vi "XML_Get_Modbus_Items.vi"(8 "error in (no error)":errorcluster, 10 "General Settings":T1={"Communication_Type"=0, "Modbus_Type"=0, "Read_Write_Loop_Period"=-1, "TCP Settings"={"TCP_Settings_Port"=0, "TCP_Settings_IP_Timeout"=0, "TCP_Settings_IP_Slave_Address"=""}, "Serial Settings"={"Serial_Settings_Flow_Control"=0, "Serial_Settings_Baud_Rate"=0, "Serial_Settings_Parity"=0, "Serial_Settings_Resource_Name"="", "Serial_Settings_Serial_Type"=0, "Serial_Settings_Unit_ID"=0}} {"Communication_Type" items=["TCP", "Serial"]; "Modbus_Type" items=["Master", "Slave"]; "Serial Settings"."Serial_Settings_Flow_Control" items=["None", "XONXOFF", "RTSCTS", "XONXOFFANDRTSCTS", "DTRDSR", "XONXOFFANDDTRDSR"]; "Serial Settings"."Serial_Settings_Parity" items=["None", "Odd", "Even"]; "Serial Settings"."Serial_Settings_Serial_Type" items=["RTU", "ASCII"]}, 11 "reference out":refnum<k24>) -> (0 "error out":errorcluster, 2 "Array":T7[](array[typedef]), 3 "reference out":refnum<k24>)   [LabVIEW 2014, in "XML_Deserializer.lvlib"]
uses:
  XML_Deserializer.lvlib
  C:/Users/vruault.AMER/Desktop/Source code/XML Deserializer/XML VIs/API/Sub-VIs/Modbus_CD_XML.dll
  Modbus_CD_XML.dll
  Controls/Modbus_Items.ctl
  Controls/Modbus_Item_Type.ctl
  Controls/Modbus_General_Settings.ctl
  Controls/Modbus_Communication_Type.ctl
  Controls/Modbus_Type.ctl
  Controls/Modbus_Serial_Settings_Flow_Control.ctl
  Controls/Modbus_Serial_Settings_Parity.ctl
  Controls/Modbus_Serial_Settings_Serial_Type.ctl
  Shared/Modbus Shared.lvlib
  System Explorer/Modbus System Explorer.lvlib
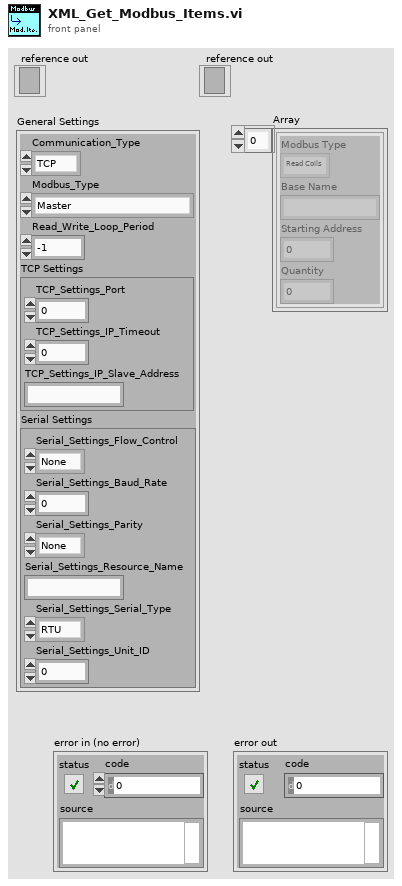
[diagram p1: front panel]
types:
  T1 = typedef "Modbus Shared.lvlib/Modbus_General_Settings.ctl" = cluster{"Communication_Type":T2, "Modbus_Type":T3, "Read_Write_Loop_Period":i64, "TCP Settings":cluster{"TCP_Settings_Port":u16, "TCP_Settings_IP_Timeout":u32, "TCP_Settings_IP_Slave_Address":string}, "Serial Settings":cluster{"Serial_Settings_Flow_Control":T4, "Serial_Settings_Baud_Rate":u32, "Serial_Settings_Parity":T5, "Serial_Settings_Resource_Name":string, "Serial_Settings_Serial_Type":T6, "Serial_Settings_Unit_ID":u8}}
  T2 = typedef "Modbus Shared.lvlib/Modbus_Communication_Type.ctl" = i32
  T3 = typedef "Modbus Shared.lvlib/Modbus_Type.ctl" = i32
  T4 = typedef "Modbus Shared.lvlib/Modbus_Serial_Settings_Flow_Control.ctl" = i32
  T5 = typedef "Modbus Shared.lvlib/Modbus_Serial_Settings_Parity.ctl" = i32
  T6 = typedef "Modbus Shared.lvlib/Modbus_Serial_Settings_Serial_Type.ctl" = i32
  T7 = typedef "Modbus Shared.lvlib/Modbus_Items.ctl" = cluster{"Modbus Type":T8, "Base Name":string, "Starting Address":u16, "Quantity":u16}
  T8 = typedef "Modbus Shared.lvlib/Modbus_Item_Type.ctl" = enum16{"Read Coils", "Read Discrete Inputs", "Read Holding Registers", "Read Input Registers", "Write Multiple Coils", "Write Multiple Holding Registers", "Write Single Coil", "Write Single Holding Register", "Write Multiple Discrete Inputs", "Write Multiple Input Registers"}
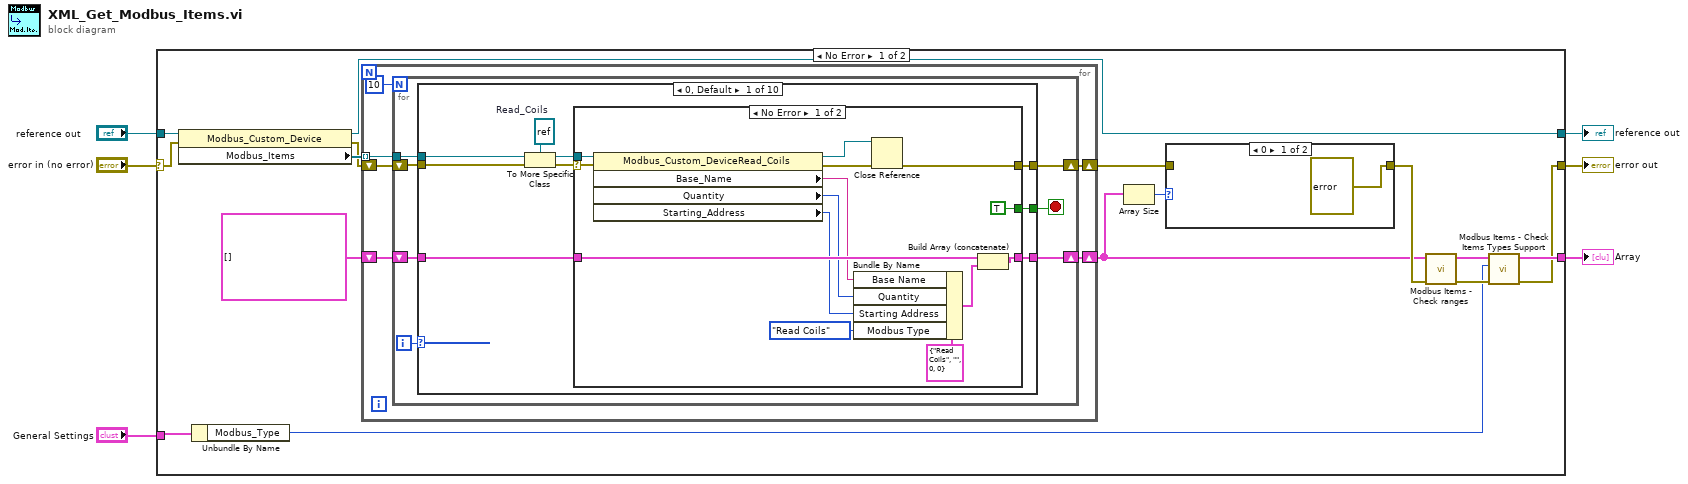
[diagram p0: block diagram]
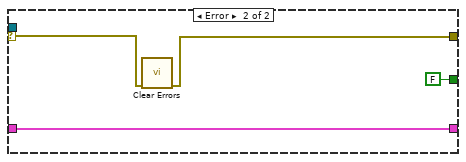
[diagram p3: hidden frame]
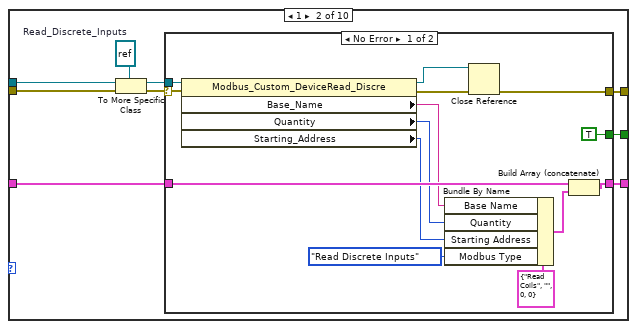
[diagram p4: hidden frame]
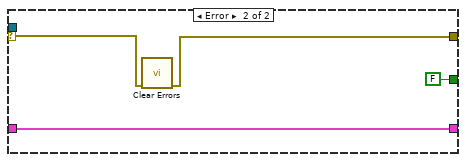
[diagram p5: hidden frame]
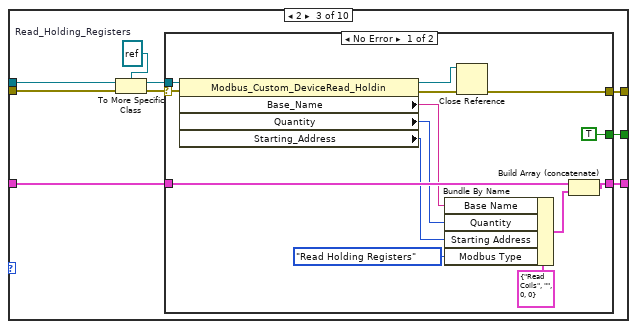
[diagram p6: hidden frame]
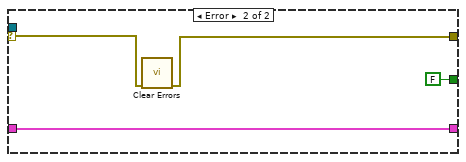
[diagram p7: hidden frame]
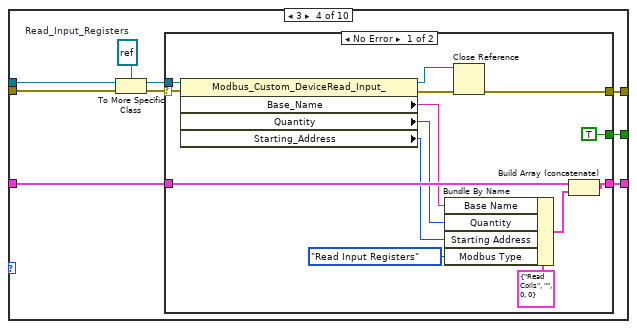
[diagram p8: hidden frame]
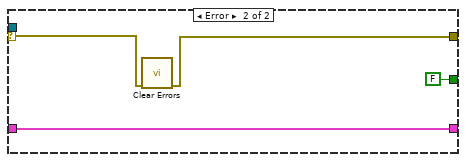
[diagram p9: hidden frame]
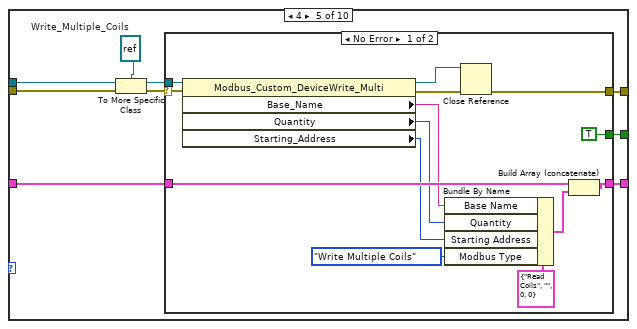
[diagram p10: hidden frame]
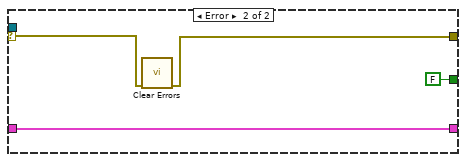
[diagram p11: hidden frame]
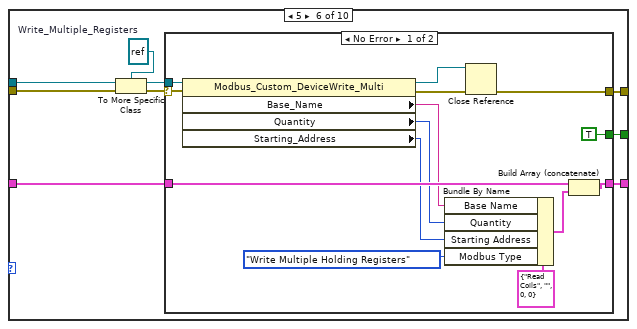
[diagram p12: hidden frame]
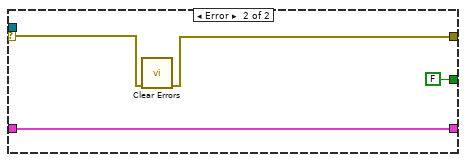
[diagram p13: hidden frame]
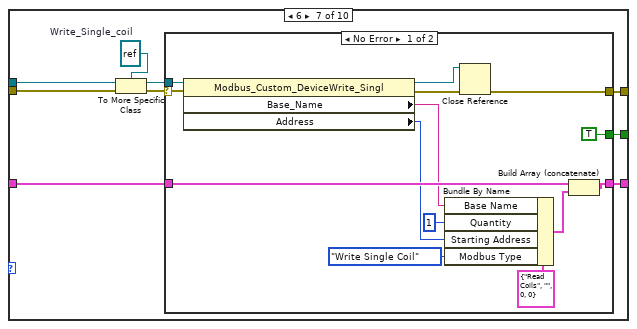
[diagram p14: hidden frame]
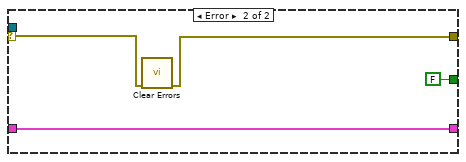
[diagram p15: hidden frame]
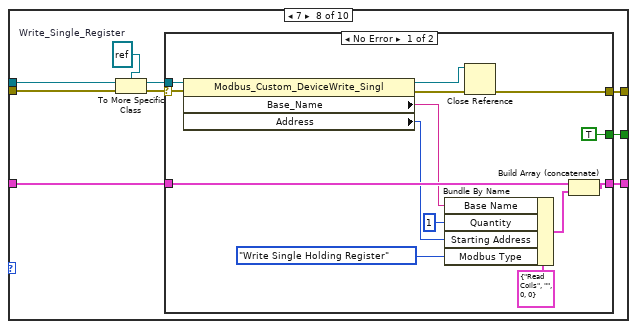
[diagram p16: hidden frame]
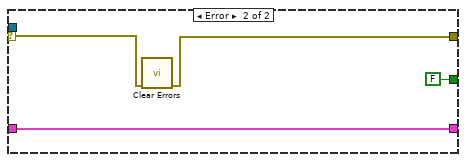
[diagram p17: hidden frame]
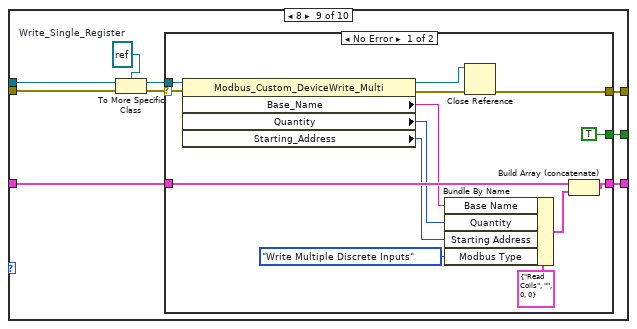
[diagram p18: hidden frame]
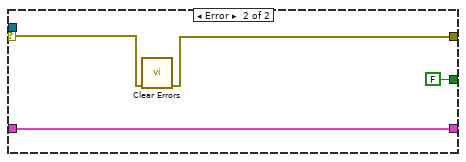
[diagram p19: hidden frame]
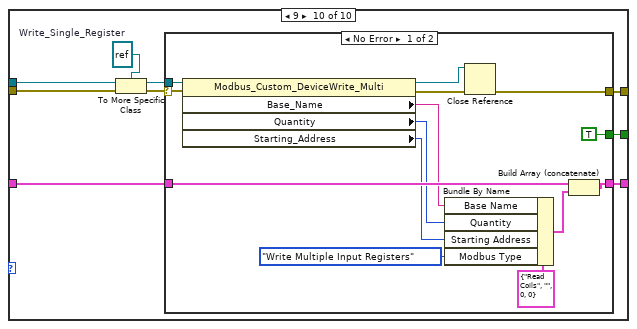
[diagram p20: hidden frame]
diagram:
  n1 = case shown="No Error" "error in (no error)" {
    selector: "error in (no error)" -> [w18 w310]
    tunnel: [w10 T7[] []] -> w2
    tunnel: [w9 w310] -> w3
    tunnel: "reference out" -> [w19 w308]
    tunnel: [w17 w308] -> w6
    tunnel: "General Settings" -> [w8 _]
    frame No Error {
      n2 = property class="Modbus_Custom_Device"(reference=w19, error in=w18) -> (reference out=w17:refnum<k24>, error out=w20:errorcluster, "Modbus_Items"=w22:refnum<k24>[])
      n3 = Unbundle By Name(w8) -> ("Modbus_Type"=w7:T3)
      n4 = for {
        tunnel: w22 -> [w30] mode=indexing
        shift-right: [w28] -> w13
        shift-left: T7[] [] -> [w29]
        shift-right: [w27] -> w15
        shift-left: w20 -> [w26]
        n5 = for {
          N: 10 -> [_]
          tunnel: w30 -> [w37]
          shift-right: [w33] -> w28
          shift-left: w29 -> [w34]
          shift-right: [w32] -> w27
          shift-left: w26 -> [w36]
          i -> [w35]
          stop <- w31 stop-if-true
          n6 = case shown="0, Default" w35 {
            tunnel: w37 -> [w46 w73 w100 w127 w154 w181 w208 w235 w262 w289]
            tunnel: w36 -> [w45 w72 w99 w126 w153 w180 w207 w234 w261 w288]
            tunnel: w34 -> [w41 w69 w96 w123 w150 w177 w204 w231 w258 w285]
            tunnel: [w40 w68 w95 w122 w149 w176 w203 w230 w257 w284] -> w33
            tunnel: [w39 w67 w94 w121 w148 w175 w202 w229 w256 w283] -> w32
            tunnel: [w38 w66 w93 w120 w147 w174 w201 w228 w255 w282] -> w31
            frame 0, Default {
              w44 = refnum<k24> refnum  # Read_Coils
              n7 = To More Specific Class(target class=w44, reference=w46, error in=w45) -> (specific class reference=w43:refnum<k24>, error out=w42:errorcluster)
              n8 = case shown="No Error" w42 {
                selector: w42 -> [w59 w64]
                tunnel: w43 -> [w60 _]
                tunnel: w41 -> [w57 w61]
                tunnel: [w56 w61] -> w40
                tunnel: [w48 w62] -> w39
                tunnel: [TRUE FALSE] -> w38
                frame No Error {
                  n9 = property class="Modbus_Custom_DeviceRead_Coils"(reference=w60, error in=w59) -> (reference out=w47:refnum<k24>, error out=w49:errorcluster, "Base_Name"=w52:string, "Quantity"=w51:u16, "Starting_Address"=w50:u16)
                  n10 = Bundle By Name(cluster=T7 {"Modbus Type"=enum."Read Coils", "Base Name"="", "Starting Address"=0, "Quantity"=0} ("Modbus Items"), "Base Name"=w52, "Quantity"=w51, "Starting Address"=w50, "Modbus Type"=Modbus_Item_Type."Read Coils") -> (w55:T7)
                  n11 = Close Reference(reference=w47, error in (no error)=w49) -> (error out=w48:errorcluster)
                  n12 = Build Array (concatenate)(w57, w55) -> (w56:T7[])
                }
                frame Error {
                  n13 = call <vilib>:"Clear Errors.vi"("error in (no error)"=w64) -> ("error out"=w62:errorcluster)  [unwired: 5 in, 1 out]
                }
              }
            }
            frame 1 {
              w65 = refnum<k24> refnum  # Read_Discrete_Inputs
              n14 = To More Specific Class(target class=w65, reference=w73, error in=w72) -> (specific class reference=w71:refnum<k24>, error out=w70:errorcluster)
              n15 = case shown="No Error" w70 {
                selector: w70 -> [w86 w91]
                tunnel: w71 -> [w87 _]
                tunnel: w69 -> [w84 w88]
                tunnel: [w83 w88] -> w68
                tunnel: [w74 w89] -> w67
                tunnel: [TRUE FALSE] -> w66
                frame No Error {
                  n16 = property class="Modbus_Custom_DeviceRead_Discre"(reference=w87, error in=w86) -> (reference out=w76:refnum<k24>, error out=w75:errorcluster, "Base_Name"=w79:string, "Quantity"=w78:u16, "Starting_Address"=w77:u16)
                  n17 = Bundle By Name(cluster=T7 {"Modbus Type"=enum."Read Coils", "Base Name"="", "Starting Address"=0, "Quantity"=0} ("Modbus Items"), "Base Name"=w79, "Quantity"=w78, "Starting Address"=w77, "Modbus Type"=Modbus_Item_Type."Read Discrete Inputs") -> (w82:T7)
                  n18 = Close Reference(reference=w76, error in (no error)=w75) -> (error out=w74:errorcluster)
                  n19 = Build Array (concatenate)(w84, w82) -> (w83:T7[])
                }
                frame Error {
                  n20 = call <vilib>:"Clear Errors.vi"("error in (no error)"=w91) -> ("error out"=w89:errorcluster)  [unwired: 5 in, 1 out]
                }
              }
            }
            frame 2 {
              w92 = refnum<k24> refnum  # Read_Holding_Registers
              n21 = To More Specific Class(target class=w92, reference=w100, error in=w99) -> (specific class reference=w98:refnum<k24>, error out=w97:errorcluster)
              n22 = case shown="No Error" w97 {
                selector: w97 -> [w113 w118]
                tunnel: w98 -> [w114 _]
                tunnel: w96 -> [w111 w115]
                tunnel: [w110 w115] -> w95
                tunnel: [w101 w116] -> w94
                tunnel: [TRUE FALSE] -> w93
                frame No Error {
                  n23 = property class="Modbus_Custom_DeviceRead_Holdin"(reference=w114, error in=w113) -> (reference out=w103:refnum<k24>, error out=w102:errorcluster, "Base_Name"=w106:string, "Quantity"=w105:u16, "Starting_Address"=w104:u16)
                  n24 = Bundle By Name(cluster=T7 {"Modbus Type"=enum."Read Coils", "Base Name"="", "Starting Address"=0, "Quantity"=0} ("Modbus Items"), "Base Name"=w106, "Quantity"=w105, "Starting Address"=w104, "Modbus Type"=Modbus_Item_Type."Read Holding Registers") -> (w109:T7)
                  n25 = Close Reference(reference=w103, error in (no error)=w102) -> (error out=w101:errorcluster)
                  n26 = Build Array (concatenate)(w111, w109) -> (w110:T7[])
                }
                frame Error {
                  n27 = call <vilib>:"Clear Errors.vi"("error in (no error)"=w118) -> ("error out"=w116:errorcluster)  [unwired: 5 in, 1 out]
                }
              }
            }
            frame 3 {
              w119 = refnum<k24> refnum  # Read_Input_Registers
              n28 = To More Specific Class(target class=w119, reference=w127, error in=w126) -> (specific class reference=w125:refnum<k24>, error out=w124:errorcluster)
              n29 = case shown="No Error" w124 {
                selector: w124 -> [w140 w145]
                tunnel: w125 -> [w141 _]
                tunnel: w123 -> [w138 w142]
                tunnel: [w137 w142] -> w122
                tunnel: [w128 w143] -> w121
                tunnel: [TRUE FALSE] -> w120
                frame No Error {
                  n30 = property class="Modbus_Custom_DeviceRead_Input_"(reference=w141, error in=w140) -> (reference out=w130:refnum<k24>, error out=w129:errorcluster, "Base_Name"=w133:string, "Quantity"=w132:u16, "Starting_Address"=w131:u16)
                  n31 = Bundle By Name(cluster=T7 {"Modbus Type"=enum."Read Coils", "Base Name"="", "Starting Address"=0, "Quantity"=0} ("Modbus Items"), "Base Name"=w133, "Quantity"=w132, "Starting Address"=w131, "Modbus Type"=Modbus_Item_Type."Read Input Registers") -> (w136:T7)
                  n32 = Close Reference(reference=w130, error in (no error)=w129) -> (error out=w128:errorcluster)
                  n33 = Build Array (concatenate)(w138, w136) -> (w137:T7[])
                }
                frame Error {
                  n34 = call <vilib>:"Clear Errors.vi"("error in (no error)"=w145) -> ("error out"=w143:errorcluster)  [unwired: 5 in, 1 out]
                }
              }
            }
            frame 4 {
              w146 = refnum<k24> refnum  # Write_Multiple_Coils
              n35 = To More Specific Class(target class=w146, reference=w154, error in=w153) -> (specific class reference=w152:refnum<k24>, error out=w151:errorcluster)
              n36 = case shown="No Error" w151 {
                selector: w151 -> [w167 w172]
                tunnel: w152 -> [w168 _]
                tunnel: w150 -> [w165 w169]
                tunnel: [w164 w169] -> w149
                tunnel: [w156 w170] -> w148
                tunnel: [TRUE FALSE] -> w147
                frame No Error {
                  n37 = property class="Modbus_Custom_DeviceWrite_Multi"(reference=w168, error in=w167) -> (reference out=w155:refnum<k24>, error out=w157:errorcluster, "Base_Name"=w160:string, "Quantity"=w159:u16, "Starting_Address"=w158:u16)
                  n38 = Bundle By Name(cluster=T7 {"Modbus Type"=enum."Read Coils", "Base Name"="", "Starting Address"=0, "Quantity"=0} ("Modbus Items"), "Base Name"=w160, "Quantity"=w159, "Starting Address"=w158, "Modbus Type"=Modbus_Item_Type."Write Multiple Coils") -> (w163:T7)
                  n39 = Close Reference(reference=w155, error in (no error)=w157) -> (error out=w156:errorcluster)
                  n40 = Build Array (concatenate)(w165, w163) -> (w164:T7[])
                }
                frame Error {
                  n41 = call <vilib>:"Clear Errors.vi"("error in (no error)"=w172) -> ("error out"=w170:errorcluster)  [unwired: 5 in, 1 out]
                }
              }
            }
            frame 5 {
              w173 = refnum<k24> refnum  # Write_Multiple_Registers
              n42 = To More Specific Class(target class=w173, reference=w181, error in=w180) -> (specific class reference=w179:refnum<k24>, error out=w178:errorcluster)
              n43 = case shown="No Error" w178 {
                selector: w178 -> [w194 w199]
                tunnel: w179 -> [w195 _]
                tunnel: w177 -> [w192 w196]
                tunnel: [w191 w196] -> w176
                tunnel: [w182 w197] -> w175
                tunnel: [TRUE FALSE] -> w174
                frame No Error {
                  n44 = property class="Modbus_Custom_DeviceWrite_Multi"(reference=w195, error in=w194) -> (reference out=w183:refnum<k24>, error out=w184:errorcluster, "Base_Name"=w187:string, "Quantity"=w186:u16, "Starting_Address"=w185:u16)
                  n45 = Bundle By Name(cluster=T7 {"Modbus Type"=enum."Read Coils", "Base Name"="", "Starting Address"=0, "Quantity"=0} ("Modbus Items"), "Base Name"=w187, "Quantity"=w186, "Starting Address"=w185, "Modbus Type"=Modbus_Item_Type."Write Multiple Holding Registers") -> (w190:T7)
                  n46 = Close Reference(reference=w183, error in (no error)=w184) -> (error out=w182:errorcluster)
                  n47 = Build Array (concatenate)(w192, w190) -> (w191:T7[])
                }
                frame Error {
                  n48 = call <vilib>:"Clear Errors.vi"("error in (no error)"=w199) -> ("error out"=w197:errorcluster)  [unwired: 5 in, 1 out]
                }
              }
            }
            frame 6 {
              w200 = refnum<k24> refnum  # Write_Single_coil
              n49 = To More Specific Class(target class=w200, reference=w208, error in=w207) -> (specific class reference=w206:refnum<k24>, error out=w205:errorcluster)
              n50 = case shown="No Error" w205 {
                selector: w205 -> [w221 w226]
                tunnel: w206 -> [w222 _]
                tunnel: w204 -> [w219 w223]
                tunnel: [w218 w223] -> w203
                tunnel: [w209 w224] -> w202
                tunnel: [TRUE FALSE] -> w201
                frame No Error {
                  n51 = property class="Modbus_Custom_DeviceWrite_Singl"(reference=w222, error in=w221) -> (reference out=w211:refnum<k24>, error out=w210:errorcluster, "Base_Name"=w214:string, "Address"=w213:u16)
                  n52 = Bundle By Name(cluster=T7 {"Modbus Type"=enum."Read Coils", "Base Name"="", "Starting Address"=0, "Quantity"=0} ("Modbus Items"), "Base Name"=w214, "Quantity"=u16 1, "Starting Address"=w213, "Modbus Type"=Modbus_Item_Type."Write Single Coil") -> (w217:T7)
                  n53 = Close Reference(reference=w211, error in (no error)=w210) -> (error out=w209:errorcluster)
                  n54 = Build Array (concatenate)(w219, w217) -> (w218:T7[])
                }
                frame Error {
                  n55 = call <vilib>:"Clear Errors.vi"("error in (no error)"=w226) -> ("error out"=w224:errorcluster)  [unwired: 5 in, 1 out]
                }
              }
            }
            frame 7 {
              w227 = refnum<k24> refnum  # Write_Single_Register
              n56 = To More Specific Class(target class=w227, reference=w235, error in=w234) -> (specific class reference=w233:refnum<k24>, error out=w232:errorcluster)
              n57 = case shown="No Error" w232 {
                selector: w232 -> [w248 w253]
                tunnel: w233 -> [w249 _]
                tunnel: w231 -> [w246 w250]
                tunnel: [w245 w250] -> w230
                tunnel: [w236 w251] -> w229
                tunnel: [TRUE FALSE] -> w228
                frame No Error {
                  n58 = property class="Modbus_Custom_DeviceWrite_Singl"(reference=w249, error in=w248) -> (reference out=w238:refnum<k24>, error out=w237:errorcluster, "Base_Name"=w241:string, "Address"=w240:u16)
                  n59 = Bundle By Name(cluster=T7 {"Modbus Type"=enum."Read Coils", "Base Name"="", "Starting Address"=0, "Quantity"=0} ("Modbus Items"), "Base Name"=w241, "Quantity"=u16 1, "Starting Address"=w240, "Modbus Type"=Modbus_Item_Type."Write Single Holding Register") -> (w244:T7)
                  n60 = Close Reference(reference=w238, error in (no error)=w237) -> (error out=w236:errorcluster)
                  n61 = Build Array (concatenate)(w246, w244) -> (w245:T7[])
                }
                frame Error {
                  n62 = call <vilib>:"Clear Errors.vi"("error in (no error)"=w253) -> ("error out"=w251:errorcluster)  [unwired: 5 in, 1 out]
                }
              }
            }
            frame 8 {
              w254 = refnum<k24> refnum  # Write_Single_Register
              n63 = To More Specific Class(target class=w254, reference=w262, error in=w261) -> (specific class reference=w260:refnum<k24>, error out=w259:errorcluster)
              n64 = case shown="No Error" w259 {
                selector: w259 -> [w275 w280]
                tunnel: w260 -> [w276 _]
                tunnel: w258 -> [w273 w277]
                tunnel: [w272 w277] -> w257
                tunnel: [w265 w278] -> w256
                tunnel: [TRUE FALSE] -> w255
                frame No Error {
                  n65 = property class="Modbus_Custom_DeviceWrite_Multi"(reference=w276, error in=w275) -> (reference out=w267:refnum<k24>, error out=w266:errorcluster, "Base_Name"=w268:string, "Quantity"=w263:u16, "Starting_Address"=w264:u16)
                  n66 = Bundle By Name(cluster=T7 {"Modbus Type"=enum."Read Coils", "Base Name"="", "Starting Address"=0, "Quantity"=0} ("Modbus Items"), "Base Name"=w268, "Quantity"=w263, "Starting Address"=w264, "Modbus Type"=Modbus_Item_Type."Write Multiple Discrete Inputs") -> (w271:T7)
                  n67 = Close Reference(reference=w267, error in (no error)=w266) -> (error out=w265:errorcluster)
                  n68 = Build Array (concatenate)(w273, w271) -> (w272:T7[])
                }
                frame Error {
                  n69 = call <vilib>:"Clear Errors.vi"("error in (no error)"=w280) -> ("error out"=w278:errorcluster)  [unwired: 5 in, 1 out]
                }
              }
            }
            frame 9 {
              w281 = refnum<k24> refnum  # Write_Single_Register
              n70 = To More Specific Class(target class=w281, reference=w289, error in=w288) -> (specific class reference=w287:refnum<k24>, error out=w286:errorcluster)
              n71 = case shown="No Error" w286 {
                selector: w286 -> [w302 w307]
                tunnel: w287 -> [w303 _]
                tunnel: w285 -> [w300 w304]
                tunnel: [w299 w304] -> w284
                tunnel: [w292 w305] -> w283
                tunnel: [TRUE FALSE] -> w282
                frame No Error {
                  n72 = property class="Modbus_Custom_DeviceWrite_Multi"(reference=w303, error in=w302) -> (reference out=w294:refnum<k24>, error out=w293:errorcluster, "Base_Name"=w295:string, "Quantity"=w290:u16, "Starting_Address"=w291:u16)
                  n73 = Bundle By Name(cluster=T7 {"Modbus Type"=enum."Read Coils", "Base Name"="", "Starting Address"=0, "Quantity"=0} ("Modbus Items"), "Base Name"=w295, "Quantity"=w290, "Starting Address"=w291, "Modbus Type"=Modbus_Item_Type."Write Multiple Input Registers") -> (w298:T7)
                  n74 = Close Reference(reference=w294, error in (no error)=w293) -> (error out=w292:errorcluster)
                  n75 = Build Array (concatenate)(w300, w298) -> (w299:T7[])
                }
                frame Error {
                  n76 = call <vilib>:"Clear Errors.vi"("error in (no error)"=w307) -> ("error out"=w305:errorcluster)  [unwired: 5 in, 1 out]
                }
              }
            }
          }
        }
      }
      n77 = Array Size(array=w13) -> (size(s)=w16:i32)
      n78 = case shown="0" w16 {
        tunnel: w15 -> [_ w24]
        tunnel: [errorcluster {"status"=TRUE, "code"=5003, "source"="Error in XML File: \"Modbus_Items\" tag doesn't have elements inside. At least one element is required."} ("error out") w24] -> w14
        frame 0 {
        }
        frame 1, Default {
        }
      }
      n79 = call "Modbus Items - Check ranges.vi"("error in (no error)"=w14, "Modbus Items In"=w13) -> ("error out"=w11:errorcluster, "Modbus Items Out"=w12:T7[])  [unwired: 8 in]
      n80 = call "Modbus Items - Check Items Types Support.vi"("error in (no error)"=w11, "Modbus_Type"=w7, "Modbus Items In"=w12) -> ("error out"=w9:errorcluster, "Modbus Items Out"=w10:T7[])  [unwired: 7 in]
    }
    frame Error {
    }
  }
  "reference out" <- w6
  "error out" <- w3
  "Array" <- w2
